vi "stim config negative duration warning (sub-vi).vi"(1 "entry line index (-1, no entry index)":i32=-1) -> (0 "error":errorcluster)   [LabVIEW 2021]
uses:
  type-defs/project_custom_error_codes_ring (type def).ctl
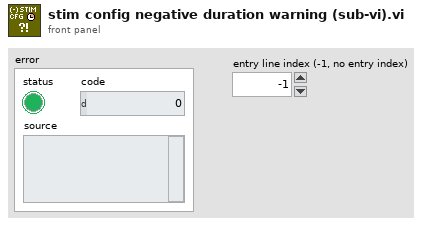
[diagram p1: front panel]
types:
  T1 = typedef "project_custom_error_codes_ring (type def).ctl" = i32
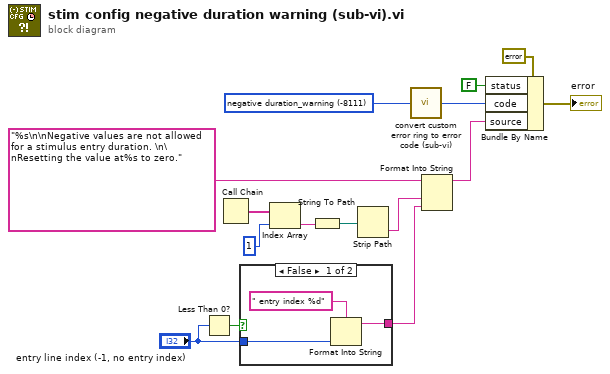
[diagram p0: block diagram]
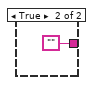
[diagram p2: hidden frame]
diagram:
  w7 = T1 -8111 items=["parse_failure"=-8001, "arduino_failure"=-8002, "manifold_config_value_error"=-8101, "odor_config_value_error"=-8102, "negative duration_warning"=-8111] ("Ring")
  n1 = Less Than 0?(x="entry line index (-1, no entry index)") -> (x < 0?=w9:bool)
  n2 = Call Chain() -> (call chain=w5:string[])
  n3 = case shown="False" w9 {
    tunnel: [w17 ""] -> w6
    tunnel: "entry line index (-1, no entry index)" -> [w16 _]
    frame False {
      n4 = Format Into String(format string=" entry index %d", w16) -> (resulting string=w17:string)  [unwired: 2 in, 1 out]
    }
    frame True {
    }
  }
  n5 = Index Array(array=w5, index=1) -> (element=w3:string)
  n6 = String To Path(string=w3) -> (path=w2:path)
  n7 = Strip Path(path=w2) -> (name=w1:string)  [unwired: 1 out]
  n8 = call "convert custom error ring to error code (sub-vi).vi"("custom error ring"=w7) -> ("error code"=w13:i32)  [unwired: 4 in]
  n9 = Format Into String(format string="%s\n\nNegative values are not allowed for a stimulus entry duration. \n\nResetting the value at%s to zero." ("source"), w1, w6) -> (resulting string=w11:string)  [unwired: 2 in, 1 out]
  n10 = Bundle By Name(cluster=errorcluster {"status"=FALSE, "code"=0, "source"=""} ("error constant"), "status"=FALSE, "code"=w13, "source"=w11) -> (→"error":errorcluster)
